vi "Read Spectrum.vi"(8 "error in (no error)":errorcluster, 11 "Spectral Processing in":refnum<class "Spectral Processing.lvclass">) -> (0 "error out":errorcluster, 2 "Spectrum":dbl[](array[numeric]), 3 "Spectral Processing out":refnum<class "Spectral Processing.lvclass">)   [LabVIEW 2014, in "Spectral Processing.lvclass"]
uses:
  Spectral Processing.lvclass
  Spectral Processing.lvclass/Spectral Processing.ctl
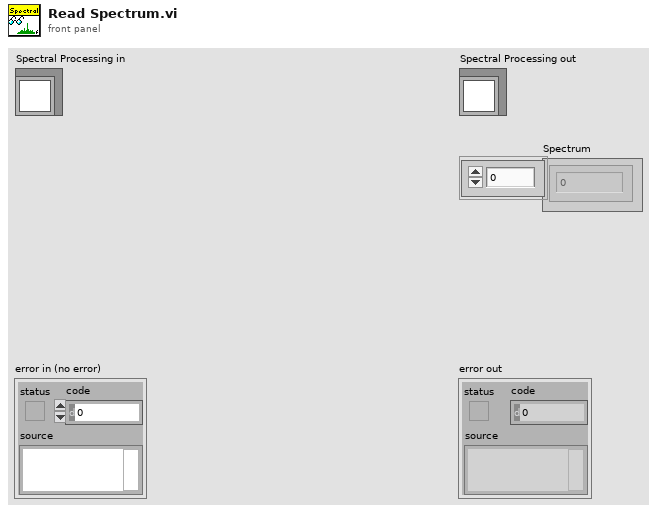
[diagram p1: front panel]
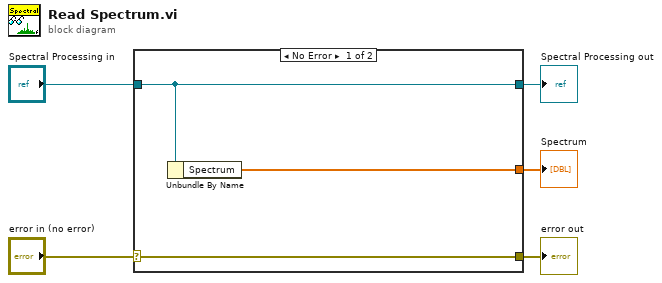
[diagram p0: block diagram]
diagram:
  n1 = case shown="No Error" "error in (no error)" {
    selector: "error in (no error)" -> [w8 w9]
    tunnel: [w8 w9] -> w4
    tunnel: [w7 w10] -> w2
    tunnel: "Spectral Processing in" -> [w7 w10]
    tunnel: [w6 _] -> w1
    frame No Error {
      n2 = Unbundle By Name(w7) -> ("Spectrum"=w6:dbl[])
    }
    frame Error {
    }
  }
  "error out" <- w4
  "Spectral Processing out" <- w2
  "Spectrum" <- w1
